vi "IsTokenInConfigList.vi"(1 "config list found?":bool, 2 "config list":string, 3 "query":string) -> (0 "in list":bool)   [LabVIEW 2017, in "Feed.lvclass"]
uses:
  <vilib>/NI_RSS/Feed/Feed.lvclass
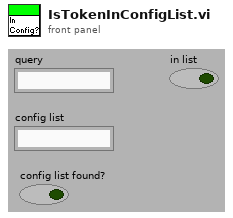
[diagram p1: front panel]
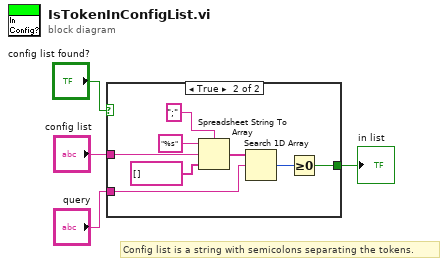
[diagram p0: block diagram]
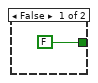
[diagram p2: hidden frame]
diagram:
  # "Config list is a string with semicolons separating the tokens."
  n1 = case shown="True" "config list found?" {
    tunnel: "config list" -> [_ w13]
    tunnel: "query" -> [_ w8]
    tunnel: [FALSE w6] -> w4
    frame False {
    }
    frame True {
      n2 = Spreadsheet String To Array(delimiter (Tab)=";", format string="%s", spreadsheet string=w13, array type (2D Dbl)=string[] []) -> (array=w9:string[])
      n3 = Search 1D Array(1D array=w9, element=w8) -> (index of element=w7:i32)  [unwired: 1 out]
      n4 = Greater Or Equal To 0?(x=w7) -> (x >= 0?=w6:bool)
    }
  }
  "in list" <- w4
